vi "IMAQController.ObjectConfig_panel.vi"(0 "object ref":refnum<vi>, 1 "IMAQDevice":string, 2 "IMAQAnalyser":string, 3 "Sequencer":string, 4 "Scanner":string) -> (7 "Device changed?":bool, 9 "Analyser changed?":bool, 11 "Sequencer changed?":bool, 13 "Scanner changed?":bool, 15 "IMAQDevice Indicator":string, 16 "IMAQAnalyser Indicator":string, 17 "Sequencer Indicator":string, 18 "Scanner Indicator":string)   [LabVIEW 2014, in "IMAQController.lvlib"]
uses:
  IMAQController.lvlib
  CSCore/CSSystem/CSSystemLib/CSSystemLib.lvlib
panel:
  in  "Cancel button":bool
  in  "OK button":bool
  out "Scanner error":bool
  out "Sequencer error":bool
  out "IMAQAnalyser error":bool
  out "IMAQDevice error":bool
  in  "Scanner button":bool
  in  "Sequencer button":bool
  in  "IMAQAnalyser button":bool
  in  "IMAQDevice button":bool
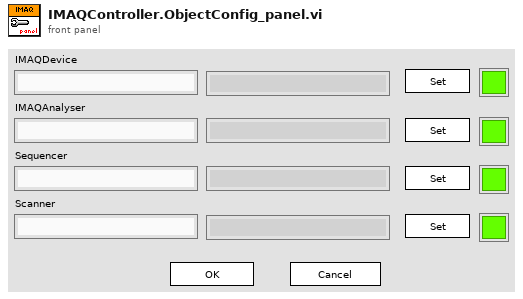
[diagram p1: front panel]
types:
  T1 = enum8{"Enabled", "Disabled", "Disabled and Grayed Out"}
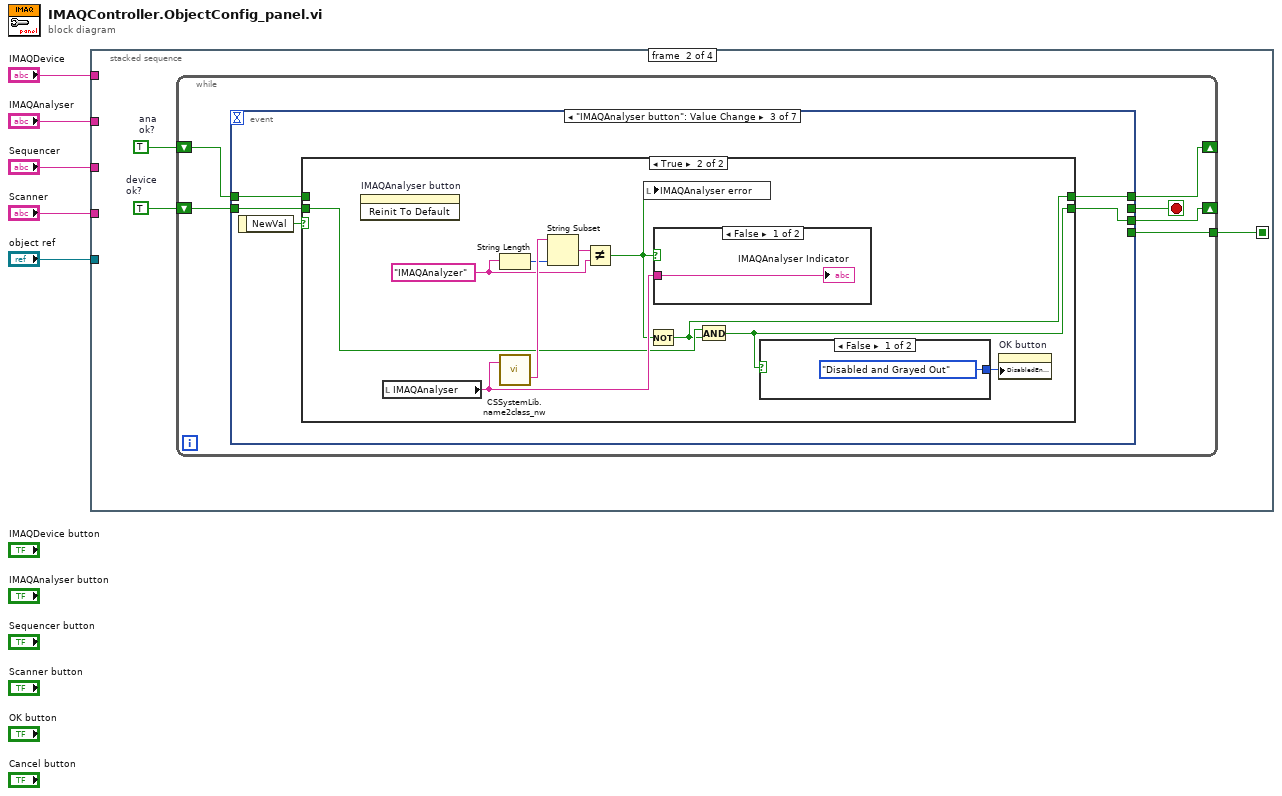
[diagram p0: block diagram]
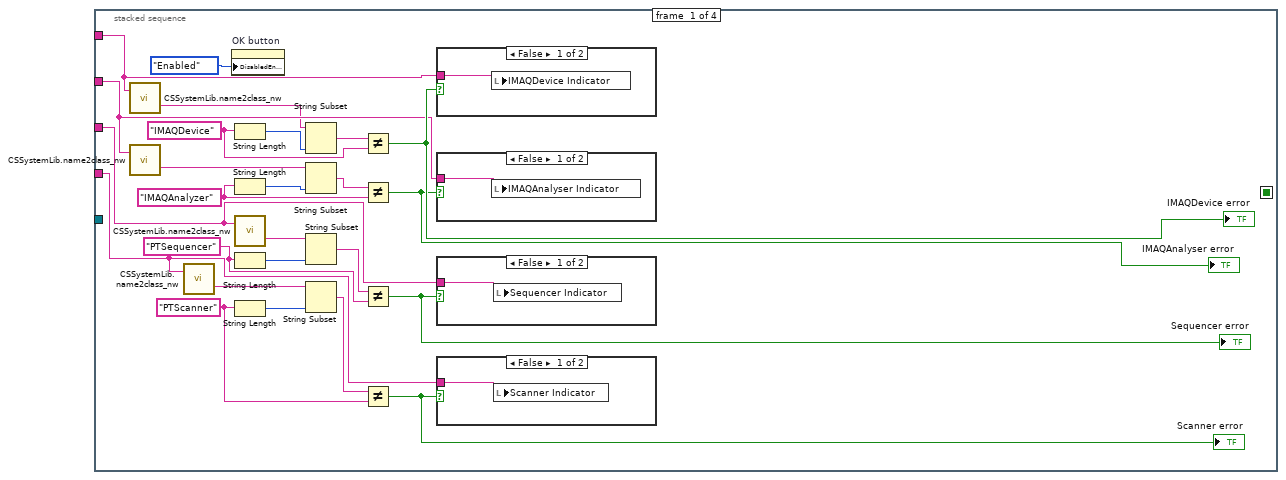
[diagram p2: hidden frame]
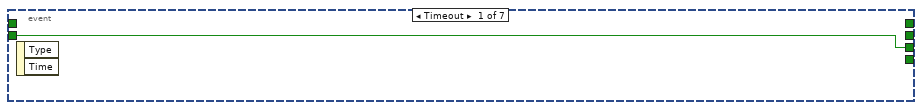
[diagram p7: hidden frame]
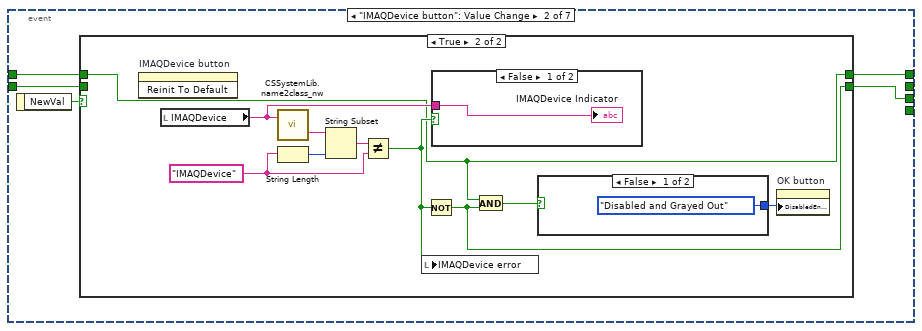
[diagram p8: hidden frame]
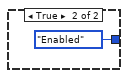
[diagram p10: hidden frame]
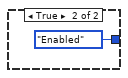
[diagram p13: hidden frame]
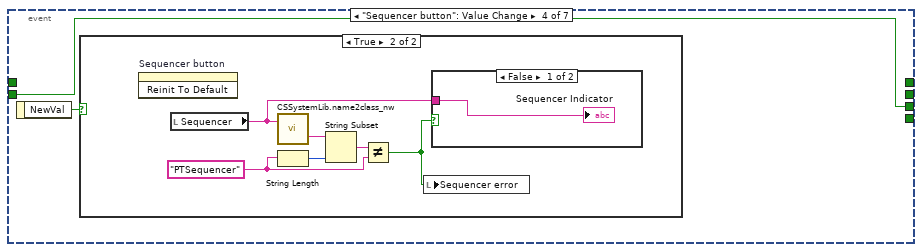
[diagram p15: hidden frame]
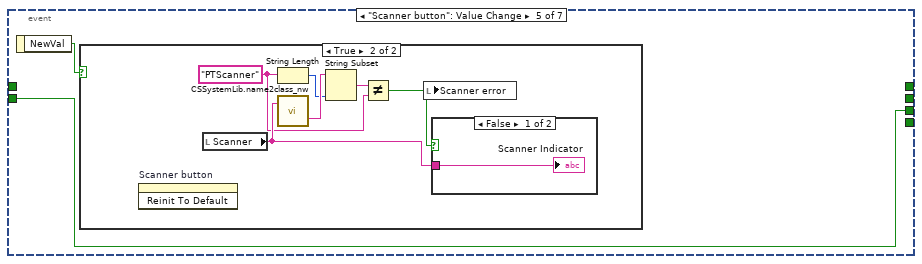
[diagram p18: hidden frame]
diagram:
  n1 = stacked-sequence {
    seq-local: [_ w37 _ _] -> [_ _ w111 _]
    tunnel: "IMAQDevice" -> [w23 _ w107 w127]
    tunnel: "IMAQAnalyser" -> [w24 _ w108 w125]
    tunnel: "Sequencer" -> [w25 _ w109 w124]
    tunnel: "Scanner" -> [w26 _ w110 w123]
    tunnel: "object ref" -> [_ _ _ _]
    frame #0 {
      w8 = "IMAQAnalyzer" ("y")
      w12 = "PTSequencer" ("y")
      w16 = "PTScanner" ("y")
      w22 = "IMAQDevice" ("y")
      n2 = call "CSSystemLib.name2class_nw.vi"("name"=w23) -> ("classID"=w20:string)  [unwired: 16 in, 2 out]
      n3 = call "CSSystemLib.name2class_nw.vi"("name"=w24) -> ("classID"=w10:string)  [unwired: 16 in, 2 out]
      n4 = call "CSSystemLib.name2class_nw.vi"("name"=w26) -> ("classID"=w18:string)  [unwired: 16 in, 2 out]
      n5 = property on="OK button" class="Bool"("DisabledEnum"=T1."Enabled" ("Disabled")) -> ()  [unwired: 2 in, 2 out]
      n6 = String Length(string=w22) -> (length=w19:i32)
      n7 = String Length(string=w8) -> (length=w7:i32)
      n8 = call "CSSystemLib.name2class_nw.vi"("name"=w25) -> ("classID"=w14:string)  [unwired: 16 in, 2 out]
      n9 = String Length(string=w12) -> (length=w11:i32)
      n10 = String Length(string=w16) -> (length=w15:i32)
      n11 = String Subset(string=w20, length (rest)=w19) -> (substring=w21:string)  [unwired: 1 in]
      n12 = String Subset(string=w10, length (rest)=w7) -> (substring=w9:string)  [unwired: 1 in]
      n13 = String Subset(string=w14, length (rest)=w11) -> (substring=w13:string)  [unwired: 1 in]
      n14 = String Subset(string=w18, length (rest)=w15) -> (substring=w17:string)  [unwired: 1 in]
      n15 = Not Equal?(x=w21, y=w22) -> (x != y?=w30:bool)
      "IMAQDevice error" <- w30
      n16 = Not Equal?(x=w9, y=w8) -> (x != y?=w29:bool)
      "IMAQAnalyser error" <- w29
      n17 = Not Equal?(x=w13, y=w12) -> (x != y?=w28:bool)
      "Sequencer error" <- w28
      n18 = Not Equal?(x=w17, y=w16) -> (x != y?=w27:bool)
      "Scanner error" <- w27
      n19 = case shown="False" w30 {
        tunnel: w23 -> [w34 _]
        frame False {
          n20 = local write "IMAQDevice Indicator"(w34) -> ()
        }
        frame True {
        }
      }
      n21 = case shown="False" w29 {
        tunnel: w24 -> [w33 _]
        frame False {
          n22 = local write "IMAQAnalyser Indicator"(w33) -> ()
        }
        frame True {
        }
      }
      n23 = case shown="False" w28 {
        tunnel: w25 -> [w32 _]
        frame False {
          n24 = local write "Sequencer Indicator"(w32) -> ()
        }
        frame True {
        }
      }
      n25 = case shown="False" w27 {
        tunnel: w26 -> [w31 _]
        frame False {
          n26 = local write "Scanner Indicator"(w31) -> ()
        }
        frame True {
        }
      }
    }
    frame #1 {
      w35 = TRUE  # ana ok?
      w36 = TRUE  # device ok?
      n27 = while {
        tunnel: [w42] -> w37
        shift-right: [w40] -> _
        shift-left: w36 -> [w41]
        shift-right: [w38] -> _
        shift-left: w35 -> [w39]
        stop <- w43 stop-if-true
        n28 = event shown="[2] \"IMAQAnalyser button\": Value Change" {
          selector: _ -> [_ _ _ _ _ _ _]
          dyn-events: _ -> [_ _ _ _ _ _ _]
          timeout: _ -> [_ _ _ _ _ _ _]
          tunnel: [_ _ _ _ _ w103 TRUE] -> w43
          tunnel: [_ _ _ _ _ w104 _] -> w42
          tunnel: w41 -> [w44 w48 w68 w85 w94 w103 w105]
          tunnel: [w44 w47 w67 w85 w94 w103 w105] -> w40
          tunnel: w39 -> [_ w46 w65 _ _ _ _]
          tunnel: [_ w45 w66 _ _ _ _] -> w38
          event Timeout {
            n29 = event-data() -> ()  [unwired: 1 in, 2 out]
          }
          event "IMAQDevice button": Value Change {
            n30 = event-data() -> ("NewVal"=w49:bool)  [unwired: 1 in]
            n31 = case shown="True" w49 {
              tunnel: w48 -> [w51 _]
              tunnel: [w51 w52] -> w47
              tunnel: w46 -> [w50 w53]
              tunnel: [w50 w53] -> w45
              frame False {
              }
              frame True {
                w58 = "IMAQDevice" ("y")
                n32 = invoke on="IMAQDevice button" class="Bool" method="Reinit To Default"() -> ()  [unwired: 3 in, 3 out]
                n33 = local read "IMAQDevice"() -> (w61:string)
                n34 = call "CSSystemLib.name2class_nw.vi"("name"=w61) -> ("classID"=w60:string)  [unwired: 16 in, 2 out]
                n35 = String Length(string=w58) -> (length=w57:i32)
                n36 = String Subset(string=w60, length (rest)=w57) -> (substring=w59:string)  [unwired: 1 in]
                n37 = Not Equal?(x=w59, y=w58) -> (x != y?=w56:bool)
                n38 = local write "IMAQDevice error"(w56) -> ()
                n39 = Not(x=w56) -> (.not. x?=w52:bool)
                n40 = case shown="False" w56 {
                  tunnel: w61 -> [w64 _]
                  frame False {
                    "IMAQDevice Indicator" <- w64
                  }
                  frame True {
                  }
                }
                n41 = And(x=w53, y=w52) -> (x .and. y?=w55:bool)
                n42 = case shown="False" w55 {
                  tunnel: [T1."Disabled and Grayed Out" ("Disabled") T1."Enabled" ("Disabled")] -> w54
                  frame False {
                  }
                  frame True {
                  }
                }
                n43 = property on="OK button" class="Bool"("DisabledEnum"=w54) -> ()  [unwired: 2 in, 2 out]
              }
            }
          }
          event "IMAQAnalyser button": Value Change {
            n44 = event-data() -> ("NewVal"=w69:bool)  [unwired: 1 in]
            n45 = case shown="True" w69 {
              tunnel: w68 -> [w71 w75]
              tunnel: [w71 w74] -> w67
              tunnel: [w70 w72] -> w66
              tunnel: w65 -> [w70 _]
              frame False {
              }
              frame True {
                w78 = "IMAQAnalyzer" ("y")
                n46 = invoke on="IMAQAnalyser button" class="Bool" method="Reinit To Default"() -> ()  [unwired: 3 in, 3 out]
                n47 = local read "IMAQAnalyser"() -> (w81:string)
                n48 = String Length(string=w78) -> (length=w77:i32)
                n49 = call "CSSystemLib.name2class_nw.vi"("name"=w81) -> ("classID"=w80:string)  [unwired: 16 in, 2 out]
                n50 = String Subset(string=w80, length (rest)=w77) -> (substring=w79:string)  [unwired: 1 in]
                n51 = Not Equal?(x=w79, y=w78) -> (x != y?=w76:bool)
                n52 = local write "IMAQAnalyser error"(w76) -> ()
                n53 = Not(x=w76) -> (.not. x?=w72:bool)
                n54 = case shown="False" w76 {
                  tunnel: w81 -> [w84 _]
                  frame False {
                    "IMAQAnalyser Indicator" <- w84
                  }
                  frame True {
                  }
                }
                n55 = And(x=w75, y=w72) -> (x .and. y?=w74:bool)
                n56 = case shown="False" w74 {
                  tunnel: [T1."Disabled and Grayed Out" ("Disabled") T1."Enabled" ("Disabled")] -> w73
                  frame False {
                  }
                  frame True {
                  }
                }
                n57 = property on="OK button" class="Bool"("DisabledEnum"=w73) -> ()  [unwired: 2 in, 2 out]
              }
            }
          }
          event "Sequencer button": Value Change {
            n58 = event-data() -> ("NewVal"=w86:bool)  [unwired: 1 in]
            n59 = case shown="True" w86 {
              frame False {
              }
              frame True {
                w88 = "PTSequencer" ("y")
                n60 = invoke on="Sequencer button" class="Bool" method="Reinit To Default"() -> ()  [unwired: 3 in, 3 out]
                n61 = local read "Sequencer"() -> (w91:string)
                n62 = call "CSSystemLib.name2class_nw.vi"("name"=w91) -> ("classID"=w90:string)  [unwired: 16 in, 2 out]
                n63 = String Length(string=w88) -> (length=w87:i32)
                n64 = String Subset(string=w90, length (rest)=w87) -> (substring=w89:string)  [unwired: 1 in]
                n65 = Not Equal?(x=w89, y=w88) -> (x != y?=w92:bool)
                n66 = local write "Sequencer error"(w92) -> ()
                n67 = case shown="False" w92 {
                  tunnel: w91 -> [w93 _]
                  frame False {
                    "Sequencer Indicator" <- w93
                  }
                  frame True {
                  }
                }
              }
            }
          }
          event "Scanner button": Value Change {
            n68 = event-data() -> ("NewVal"=w95:bool)  [unwired: 1 in]
            n69 = case shown="True" w95 {
              frame False {
              }
              frame True {
                w97 = "PTScanner" ("y")
                n70 = invoke on="Scanner button" class="Bool" method="Reinit To Default"() -> ()  [unwired: 3 in, 3 out]
                n71 = local read "Scanner"() -> (w100:string)
                n72 = String Length(string=w97) -> (length=w96:i32)
                n73 = call "CSSystemLib.name2class_nw.vi"("name"=w100) -> ("classID"=w99:string)  [unwired: 16 in, 2 out]
                n74 = String Subset(string=w99, length (rest)=w96) -> (substring=w98:string)  [unwired: 1 in]
                n75 = Not Equal?(x=w98, y=w97) -> (x != y?=w101:bool)
                n76 = local write "Scanner error"(w101) -> ()
                n77 = case shown="False" w101 {
                  tunnel: w100 -> [w102 _]
                  frame False {
                    "Scanner Indicator" <- w102
                  }
                  frame True {
                  }
                }
              }
            }
          }
          event "OK button": Value Change {
            w104 = TRUE  # ok?
            n78 = event-data() -> ()  [unwired: 1 in, 1 out]
          }
          event "Cancel button": Value Change {
            n79 = event-data() -> ()  [unwired: 1 in, 1 out]
          }
        }
      }
    }
    frame #2 {
      n80 = case shown="True" w111 {
        tunnel: w110 -> [_ w112]
        tunnel: w109 -> [_ w113]
        tunnel: w108 -> [_ w115]
        tunnel: w107 -> [_ w114]
        frame False {
        }
        frame True {
          n81 = local write "IMAQDevice Indicator"(w114) -> ()
          n82 = local write "IMAQAnalyser Indicator"(w115) -> ()
          n83 = local write "Sequencer Indicator"(w113) -> ()
          n84 = local write "Scanner Indicator"(w112) -> ()
        }
      }
    }
    frame #3 {
      n85 = local read "IMAQAnalyser Indicator"() -> (w116:string)
      n86 = local read "IMAQDevice Indicator"() -> (w126:string)
      n87 = local read "Sequencer Indicator"() -> (w121:string)
      n88 = local read "Scanner Indicator"() -> (w122:string)
      n89 = Not Equal?(x=w127, y=w126) -> (x != y?=→"Device changed?":bool)
      n90 = Not Equal?(x=w125, y=w116) -> (x != y?=→"Analyser changed?":bool)
      n91 = Not Equal?(x=w124, y=w121) -> (x != y?=→"Sequencer changed?":bool)
      n92 = Not Equal?(x=w123, y=w122) -> (x != y?=→"Scanner changed?":bool)
    }
  }
